vi "testFlushTelQueue.vi"(8 "error in (no error)":errorcluster) -> (0 "error out":errorcluster)   [LabVIEW 2018]
doc: "Test the flushTelQueue.vi."
uses:
  src/TcpServer/TcpServer.lvclass
  src/TcpServer/TcpServer.lvclass/TcpServer.ctl
  src/TcpServerTel/TcpServerTel.lvclass/TcpServerTel.ctl
  <vilib>/addons/_JKI Toolkits/Caraya/classes/Assert/Assert Equal Value_Variant.vi
  src/TcpServerTel/TcpServerTel.lvclass
  <vilib>/addons/_JKI Toolkits/Caraya/classes/Test/Test.lvclass
  <vilib>/addons/_JKI Toolkits/Caraya/classes/Assert/Assert.lvclass
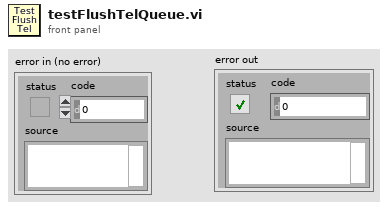
[diagram p1: front panel]
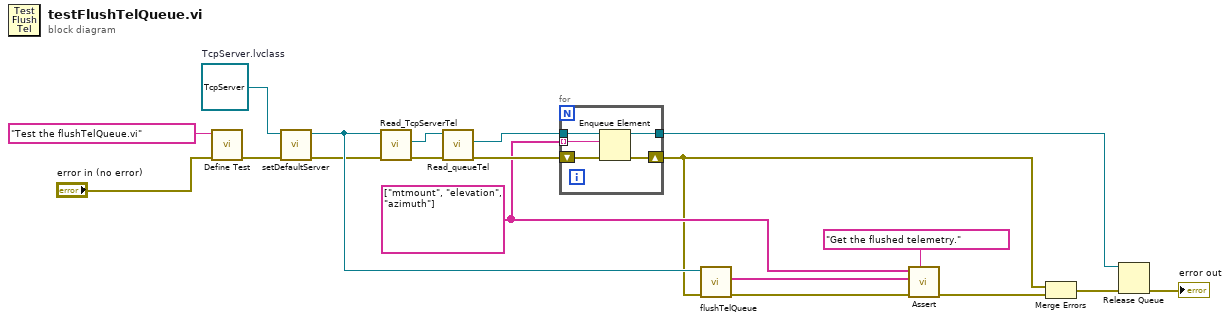
[diagram p0: block diagram]
diagram:
  w2 = string[] ["mtmount", "elevation", "azimuth"]
  w16 = refnum<class "TcpServer.lvclass"> refnum  # TcpServer.lvclass
  n1 = call <vilib>:"Define Test.vi"("error in (no error)"="error in (no error)", "Label (VI Title)"="Test the flushTelQueue.vi") -> ("error out"=w18:errorcluster)  [unwired: 9 in]
  n2 = call "setDefaultServer.vi"("error in (no error)"=w18, "TcpServer.lvclass"=w16) -> ("error out"=w5:errorcluster, "tcpServer out"=w6:refnum<class "TcpServer.lvclass">)  [unwired: 8 in]
  n3 = call "Read_TcpServerTel.vi"("error in (no error)"=w5, "TcpServer in"=w6) -> ("error out"=w12:errorcluster, "TcpServerTel.lvclass"=w13:refnum<class "TcpServerTel.lvclass">)  [unwired: 7 in, 1 out]
  n4 = call "Read_queueTel.vi"("error in (no error)"=w12, "TcpServerTel in"=w13) -> ("error out"=w9:errorcluster, "telQueueServer"=w8:refnum<queue>)  [unwired: 7 in, 1 out]
  n5 = for {
    tunnel: w8 -> [w23]
    tunnel: w2 -> [w22] mode=indexing
    tunnel: [w20] -> w7
    shift-right: [w21] -> w1
    shift-left: w9 -> [w24]
    n6 = Enqueue Element(queue=w23, element=w22, error in (no error)=w24) -> (queue out=w20:refnum<queue>, error out=w21:errorcluster)  [unwired: 1 in, 1 out]
  }
  n7 = call "flushTelQueue.vi"("error in (no error)"=w1, "TcpServer in"=w6) -> ("error out"=w4:errorcluster, "telemetry flushed"=w3:string[])  [unwired: 7 in, 1 out]
  n8 = call-poly <vilib>:"Assert.vi"("Label"="Get the flushed telemetry.", "error in (no error)"=w4, "Y"=w3, "X"=w2) -> ("error out"=w14:errorcluster)  [unwired: 7 in]
  n9 = Merge Errors(w1, w14) -> (w10:errorcluster)
  n10 = Release Queue(queue=w7, error in (no error)=w10) -> (error out=→"error out":errorcluster)  [unwired: 1 in, 2 out]
